vi "Xeryon SetDPos command.vi"(3 "Stage":string, 4 "Speed":dbl=nan, 5 "Target position":dbl) -> ()   [LabVIEW 2019]
uses:
  Xeryon Axis command.ctl
panel:
  # "//Must be dault 'NaN'"
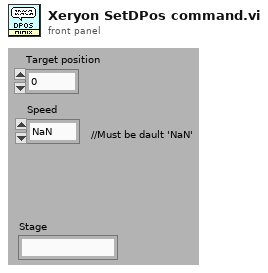
[diagram p1: front panel]
types:
  T1 = typedef "Xeryon Axis command.ctl" = cluster{"Command":enum16{"Reset", "Zero output", "Go home", "Find index", "Scan -X", "Scan +X", "Scan Stop", "Step -X", "Step +X", "Set DPOS", "Stop", "Continue", "Desired speed", "Apply settings file", "Exit", "Reset encoder", "Recover", "Save"}, "Data to send":string}
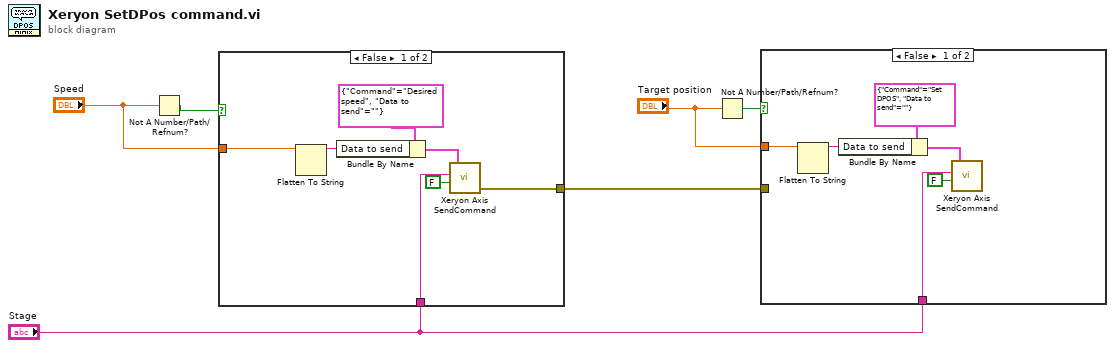
[diagram p0: block diagram]
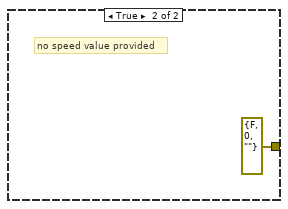
[diagram p3: hidden frame]
diagram:
  n1 = Not A Number/Path/Refnum?(number/path/refnum="Speed") -> (NaN/Path/Refnum?=w6:bool)
  n2 = case shown="False" w6 {
    tunnel: "Speed" -> [w7 _]
    tunnel: "Stage" -> [w11 _]
    tunnel: [w8 errorcluster {"status"=FALSE, "code"=0, "source"=""} ("error out")] -> w4
    frame False {
      n3 = Flatten To String(anything=w7) -> (data string=w9:string)  [unwired: 3 in, 2 out]
      n4 = Bundle By Name(cluster=T1 {"Command"=enum."Desired speed", "Data to send"=""} ("Axis Message"), "Data to send"=w9) -> (w12:T1)
      n5 = call "Xeryon Axis SendCommand.vi"("Feedback?"=FALSE, "Stage"=w11, "Axis Command"=w12) -> ("error out"=w8:errorcluster)  [unwired: 3 in]
    }
    frame True {
      # "no speed value provided"
    }
  }
  n6 = Not A Number/Path/Refnum?(number/path/refnum="Target position") -> (NaN/Path/Refnum?=w3:bool)
  n7 = case shown="False" w3 {
    tunnel: "Target position" -> [w19 _]
    tunnel: "Stage" -> [w17 _]
    tunnel: w4 -> [_ _]
    frame False {
      n8 = Flatten To String(anything=w19) -> (data string=w15:string)  [unwired: 3 in, 2 out]
      n9 = Bundle By Name(cluster=T1 {"Command"=enum."Set DPOS", "Data to send"=""} ("Axis Message"), "Data to send"=w15) -> (w18:T1)
      n10 = call "Xeryon Axis SendCommand.vi"("Feedback?"=FALSE, "Stage"=w17, "Axis Command"=w18) -> ()  [unwired: 3 in, 1 out]
    }
    frame True {
    }
  }
